vi "LSCI332 SetLoopPar.vi"(0 "VISA Rsrc":refnum<visa-resource-name>="GPIB0::12::INSTR", 5 "Boucle(1)":u32(ring) caption="Boucle" items=["Boucle 1", "Boucle 2"], 7 "Input":u32(ring) caption="Entrée" items=["A", "B"], 9 "Units":u32(ring)=1 caption="Unités du setpoint" items=["Kelvin"=1, "Celsius"=2, "Unités Capteur"=3], 11 "error in (no error)":errorcluster, 12 "PowerUp":bool caption="Contrôle actif \nau démarrage", 13 "HeatUnits":u32(ring)=1 caption="Unités du chauffage" items=["Courrant"=1, "Puissance"=2]) -> (15 "error out":errorcluster)   [LabVIEW 2019]
doc: "Ce VI écrit les paramètres limites de contrôle dans le contrôleur."
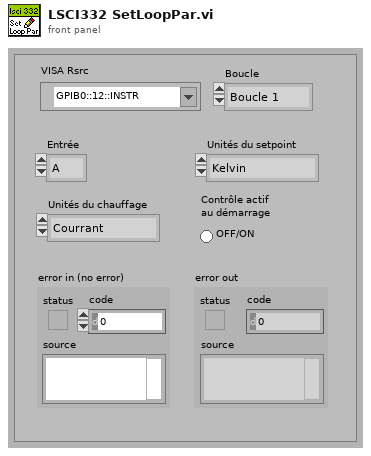
[diagram p1: front panel]
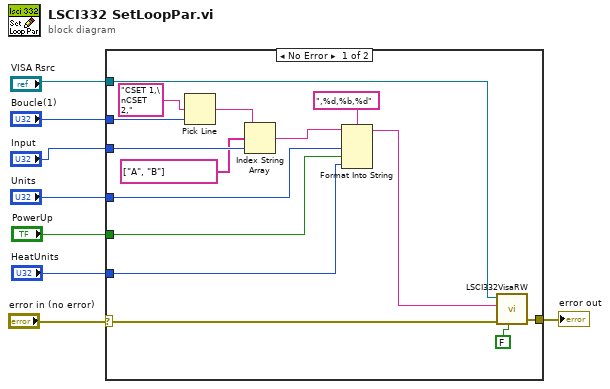
[diagram p0: block diagram]
diagram:
  n1 = case shown="No Error" "error in (no error)" {
    selector: "error in (no error)" -> [w21 w24]
    tunnel: "VISA Rsrc" -> [w23 _]
    tunnel: "Boucle(1)" -> [w18 _]
    tunnel: [w22 w24] -> w6
    tunnel: "Input" -> [w14 _]
    tunnel: "Units" -> [w15 _]
    tunnel: "PowerUp" -> [w10 _]
    tunnel: "HeatUnits" -> [w9 _]
    frame No Error {
      n2 = Pick Line(multi-line string="CSET 1,\nCSET 2,", line index=w18) -> (output string=w11:string)  [unwired: 1 in]
      n3 = Index String Array(1:w14, 2:string[] ["A", "B"] ("string array"), 3:w11) -> (0:w12:string)
      n4 = Format Into String(format string=",%d,%b,%d", initial string=w12, w15, w10, w9) -> (resulting string=w16:string)  [unwired: 1 in, 1 out]
      n5 = call <userlib>:"LSCI332VisaRW.vi"("Lecture?(T)"=FALSE, "error in (no error)"=w21, "ChaineCom"=w16, "VISA Rsrc"=w23) -> ("error out"=w22:errorcluster)  [unwired: 3 in, 3 out]
    }
    frame Error {
    }
  }
  "error out" <- w6
